vi "WaitPassTactic.vi"(6 "Tactic index in":i32, 7 "first call":bool, 8 "error in (no error)":errorcluster, 9 "Robot":refnum<class "Robot.lvclass">, 10 "Game in":refnum<class "Game.lvclass">, 11 "WaitPassTactic in":refnum<class "WaitPassTactic.lvclass">) -> (0 "error out":errorcluster, 2 "Robot out":refnum<class "Robot.lvclass">, 3 "WaitPassTactic out":refnum<class "WaitPassTactic.lvclass">)   [LabVIEW 2018, in "WaitPassTactic.lvclass"]
uses:
  WaitPassTactic.lvclass
  Robot_class/Robot.lvclass
  Game_class/Game.lvclass
  Tactic_class/Tactic.lvclass/Tactic.ctl
  Game_class/Game.lvclass/Game.ctl
  Team_class/Team.lvclass/Team.ctl
  Robot_class/Robot.lvclass/Robot.ctl
  Robot_class/tactics.ctl
  Robot_class/roles.ctl
  Skillbook_class/Skillbook.lvclass/Skillbook.ctl
  Robot_class/Read role.vi
  Skillbook_class/Read WaitBallTrajSkill.vi
  Skillbook_class/Read WaitBallKickerSkill.vi
  Skillbook_class/Read WaitBallOrientSkill.vi
  Game_class/Read OffensiveTeam.vi
  Team_class/Read OffensivePlay.vi
  Tactic_class/Read Skillbook.vi
  Robot_class/Write tactic.vi
  Ally_class/Ally.lvclass
  Skillbook_class/Skillbook.lvclass
  WaitBallTrajSkill_class/WaitBallTrajSkill.lvclass
  WaitBallKickerSkill_class/WaitBallKickerSkill.lvclass
  WaitBallOrientSkill_class/WaitBallOrientSkill.lvclass
panel:
  out "x .or. y? 2":bool
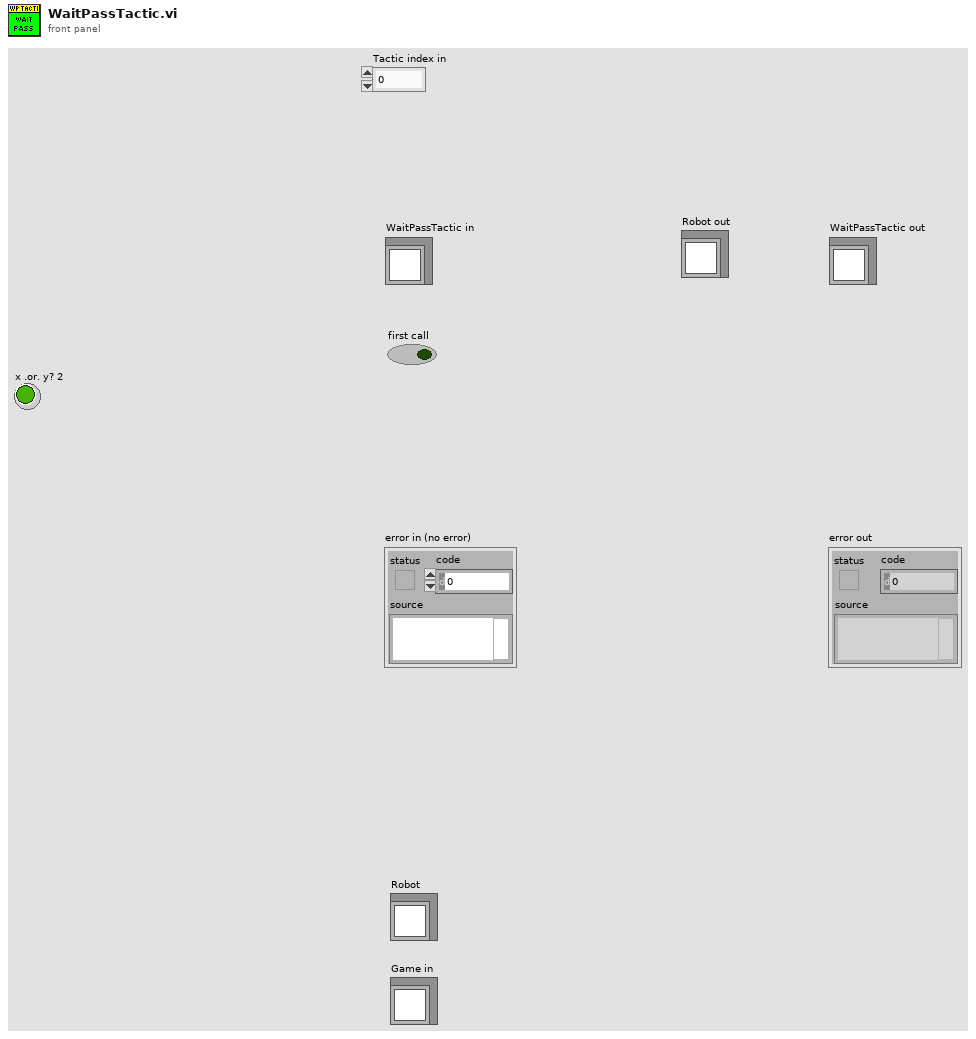
[diagram p1: front panel]
types:
  T1 = typedef "tactics.ctl" = enum16{"ReceivePassInFuturePoint", "Roller", "PrepareRollToPassRollerGoTo", "PrepareRollToPassReceiverGoTo", "WaitRoll", "PositionToRoll", "PenaltyAttacker", "PassObserver", "PenaltyDefense", "TableReceiverTactic", "Test", "DefendGoal", "Marker", "FollowAttacker", "DefendArea", "Shoot", "AttackerAimGoal", "AttackerBallOutOfField", "AttackerBlock", "AttackerStop", "Duelist", "Halt", "ZigZag", "GoTo", "Timeout", "KickToPassReceiver", "PositionToReceivePass", "WaitPass"}
  T2 = typedef "roles.ctl" = enum16{"Tabler", "TableFinalizer", "PrepareRollToPassRoller", "PrepareRollToPassReceiver", "SimplePassRoll", "SimplePassRollReceiver", "PenaltyDefense", "PreparePassReceiver 2", "PreparePassReceiver 1", "PassObserver", "Timeout", "Goto", "ZigZag", "None", "BallOutOfField", "DefenderArea", "Duelist", "AttackerStop", "FollowAttacker", "KeeperRole", "KickPenalty", "AttackerAimGoal", "AttackerBlock", "Marker", "Halt", "Shoot", "PassKicker", "PassReceiver", "TestRole", "PenaltyAttacker"}
  T3 = typedef "OffensivePlay.ctl" = enum16{"TableWithStriker", "TableWith2ndStrikerPlay", "PrepareDoublePass", "PrepareRollToPass", "SimplePass", "PreparePass", "PassToStriker", "BallOutOfField", "PassTo2ndStriker", "StopOffensive", "Prepare Penalty Enemy", "EnemyPossessionAtEnemyField", "EnemyPossesionAtOurField", "TestPlay", "PreparePenaltyAlly", "KickPenaltyAlly", "PrepareKickoffAlly", "PrepareKickoffEnemy", "IndirectEnemy", "DirectEnemy", "NormalGame", "DirectKick", "Pass", "Halt", "Timeout", "PassPlay", "PenaltyEnemy"}
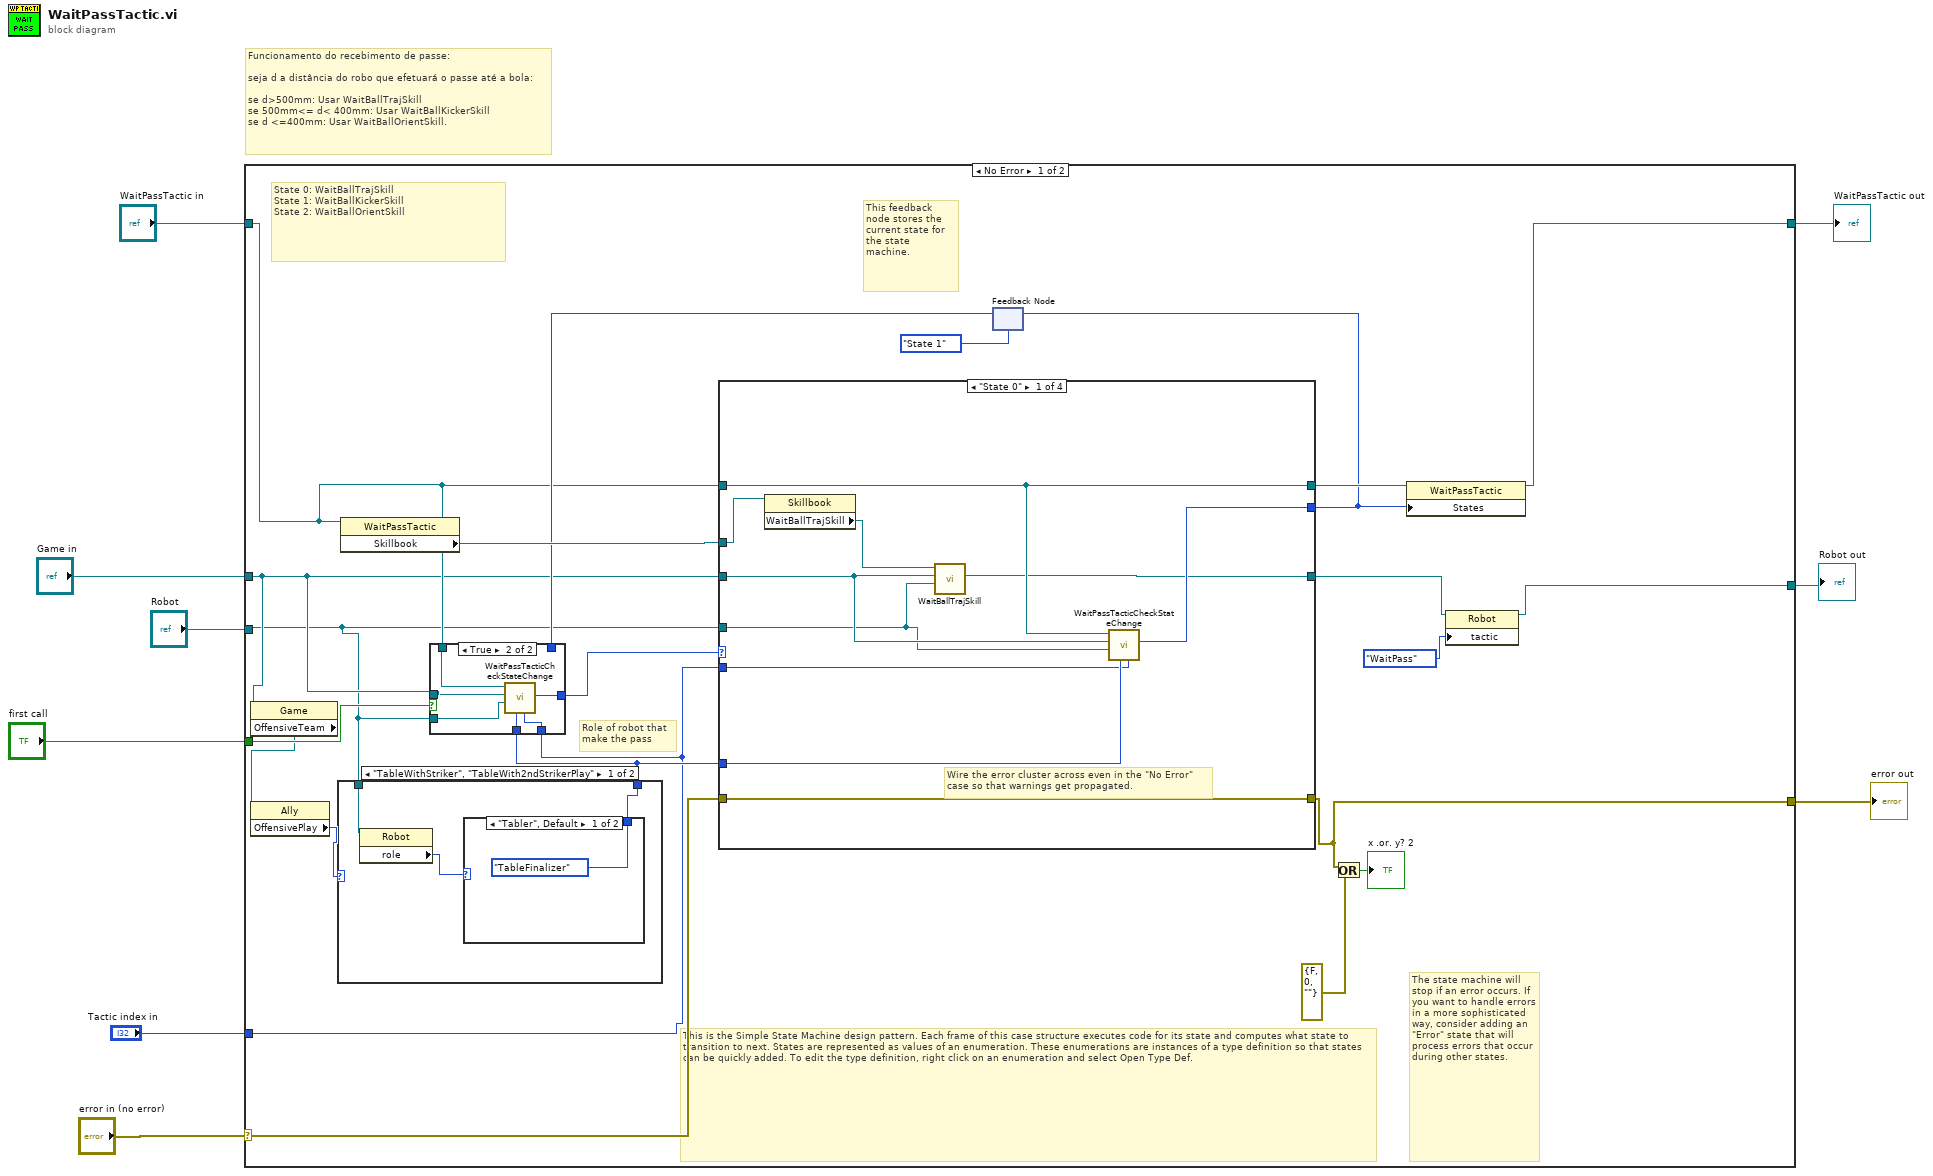
[diagram p0: block diagram]
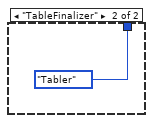
[diagram p2: hidden frame]
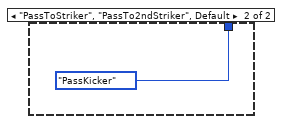
[diagram p3: hidden frame]
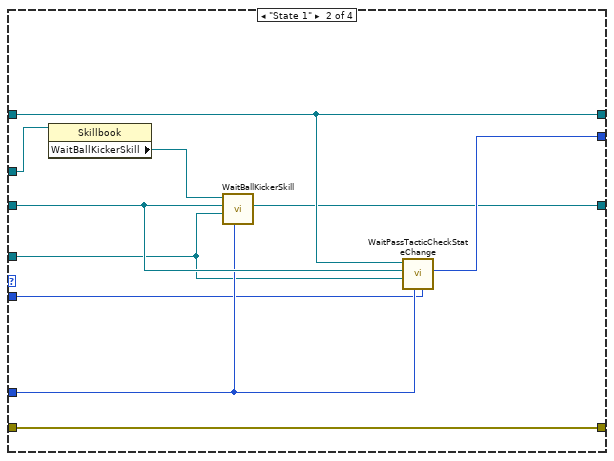
[diagram p5: hidden frame]
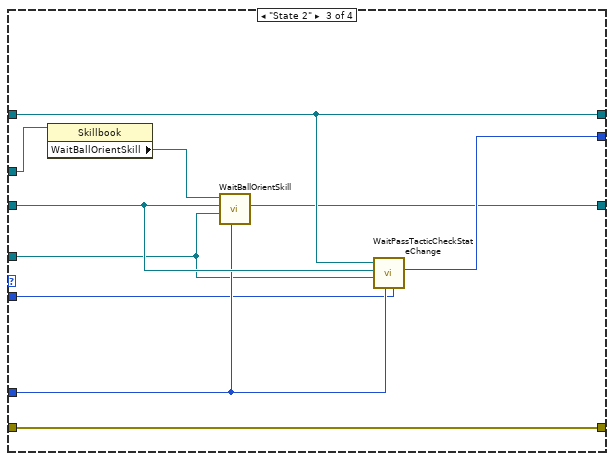
[diagram p6: hidden frame]
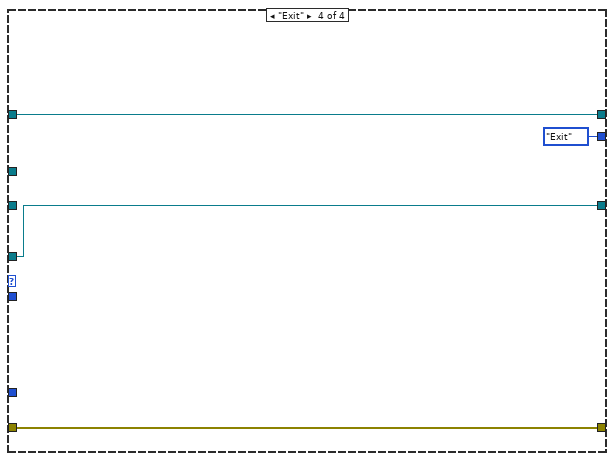
[diagram p7: hidden frame]
diagram:
  # "Funcionamento do recebimento de passe:\n\nseja d a distância do robo que efetuará o passe até a bola:\n\nse d>500mm: Usar WaitBallTrajSkill\nse 500mm<= d< 400mm: Usar WaitBallKickerSkill\nse d <=400mm: Usar WaitBallOrientSkill."
  n1 = case shown="No Error" "error in (no error)" {
    selector: "error in (no error)" -> [w20 w81]
    tunnel: [w19 w81] -> w8
    tunnel: [w17 w80] -> w6
    tunnel: "WaitPassTactic in" -> [w22 w80]
    tunnel: "Game in" -> [w15 _]
    tunnel: "Robot" -> [w12 w79]
    tunnel: [w18 w79] -> w4
    tunnel: "first call" -> [w21 _]
    tunnel: "Tactic index in" -> [w10 _]
    frame No Error {
      # "Role of robot that\nmake the pass"
      # "State 0: WaitBallTrajSkill\nState 1: WaitBallKickerSkill\nState 2: WaitBallOrientSkill"
      # "The state machine will stop if an error occurs. If you want to handle errors in a more sophisticated way, consider adding an \"Error\" state that will process errors that occur during other states."
      # "This feedback node stores the current state for the state machine."
      # "This is the Simple State Machine design pattern. Each frame of this case structure executes code for its state and computes what state to transition to next. States are represented as values of an enumeration. These enumerations are instances of a type definition so that states can be quickly added. To edit the type definition, right click on an enumeration and select Open Type Def."
      # "Wire the error cluster across even in the \"No Error\"\ncase so that warnings get propagated."
      n2 = property class="Game"(reference=w15) -> ("OffensiveTeam"=w14:refnum<class "Ally.lvclass">)  [unwired: 1 in, 2 out]
      n3 = property class="Ally"(reference=w14) -> ("OffensivePlay"=w13:T3)  [unwired: 1 in, 2 out]
      n4 = case shown="\"TableWithStriker\", \"TableWith2ndStrikerPlay\"" w13 {
        tunnel: [w32 roles."PassKicker" ("Role ofRobotThat\nmake the pass")] -> w11
        tunnel: w12 -> [w34 _]
        frame "TableWithStriker", "TableWith2ndStrikerPlay" {
          n5 = property class="Robot"(reference=w34) -> ("role"=w33:T2)  [unwired: 1 in, 2 out]
          n6 = case shown="\"Tabler\", Default" w33 {
            tunnel: [roles."TableFinalizer" ("Role ofRobotThat\nmake the pass") roles."Tabler" ("Role ofRobotThat\nmake the pass")] -> w32
            frame "Tabler", Default {
            }
            frame "TableFinalizer" {
            }
          }
        }
        frame "PassToStriker", "PassTo2ndStriker", Default {
        }
      }
      n7 = property class="WaitPassTactic"(reference=w22) -> ("Skillbook"=w30:refnum<class "Skillbook.lvclass">)  [unwired: 1 in, 2 out]
      n8 = feedback #1(enum16{"State 0", "State 1", "State 2", "Exit"}."State 1" ("States")) -> (w28:enum16{"State 0", "State 1", "State 2", "Exit"})
      n9 = case shown="True" w21 {
        tunnel: [w38 w42] -> w27
        tunnel: w28 -> [w38 _]
        tunnel: w15 -> [_ w43]
        tunnel: w22 -> [_ w44]
        tunnel: w12 -> [_ w41]
        tunnel: w11 -> [_ w40]
        tunnel: w10 -> [_ w39]
        frame False {
        }
        frame True {
          n10 = call "WaitPassTacticCheckStateChange.vi"("Tactic index in"=w39, "Role ofRobotThat\nmake the pass"=w40, "Robot in"=w41, "Game"=w43, "WaitPassTactic in"=w44) -> ("States"=w42:enum16{"State 0", "State 1", "State 2", "Exit"})  [unwired: 4 in, 2 out]
        }
      }
      n11 = case shown="\"State 0\"" w27 {
        tunnel: w20 -> [w54 w64 w74 w78]
        tunnel: [w54 w64 w74 w78] -> w19
        tunnel: w30 -> [w53 w63 w73 _]
        tunnel: w12 -> [w47 w56 w66 w75]
        tunnel: [w49 w58 w68 w75] -> w24
        tunnel: [w51 w62 w72 w77] -> w29
        tunnel: w22 -> [w51 w62 w72 w77]
        tunnel: w15 -> [w50 w59 w69 _]
        tunnel: [w52 w61 w71 enum16{"State 0", "State 1", "State 2", "Exit"}."Exit" ("States")] -> w16
        tunnel: w11 -> [w46 w57 w67 _]
        tunnel: w10 -> [w45 w55 w65 _]
        frame "State 0" {
          n12 = property class="Skillbook"(reference=w53) -> ("WaitBallTrajSkill"=w48:refnum<class "WaitBallTrajSkill.lvclass">)  [unwired: 1 in, 2 out]
          n13 = call "WaitBallTrajSkill.vi"("Robot"=w47, "Game"=w50, "WaitBallTrajSkill in"=w48) -> ("robot out"=w49:refnum<class "Robot.lvclass">)  [unwired: 6 in, 2 out]
          n14 = call "WaitPassTacticCheckStateChange.vi"("Tactic index in"=w45, "Role ofRobotThat\nmake the pass"=w46, "Robot in"=w47, "Game"=w50, "WaitPassTactic in"=w51) -> ("States"=w52:enum16{"State 0", "State 1", "State 2", "Exit"})  [unwired: 4 in, 2 out]
        }
        frame "State 1" {
          n15 = property class="Skillbook"(reference=w63) -> ("WaitBallKickerSkill"=w60:refnum<class "WaitBallKickerSkill.lvclass">)  [unwired: 1 in, 2 out]
          n16 = call "WaitBallKickerSkill.vi"("Role ofRobotThat\nmake the pass"=w57, "Robot"=w56, "Game"=w59, "WaitBallKickerSkill in"=w60) -> ("robot out"=w58:refnum<class "Robot.lvclass">)  [unwired: 5 in, 2 out]
          n17 = call "WaitPassTacticCheckStateChange.vi"("Tactic index in"=w55, "Role ofRobotThat\nmake the pass"=w57, "Robot in"=w56, "Game"=w59, "WaitPassTactic in"=w62) -> ("States"=w61:enum16{"State 0", "State 1", "State 2", "Exit"})  [unwired: 4 in, 2 out]
        }
        frame "State 2" {
          n18 = property class="Skillbook"(reference=w73) -> ("WaitBallOrientSkill"=w70:refnum<class "WaitBallOrientSkill.lvclass">)  [unwired: 1 in, 2 out]
          n19 = call "WaitBallOrientSkill.vi"("Role ofRobotThat\nmake the pass"=w67, "Robot"=w66, "Game"=w69, "WaitBallOrientSkill in"=w70) -> ("robot out"=w68:refnum<class "Robot.lvclass">)  [unwired: 5 in, 2 out]
          n20 = call "WaitPassTacticCheckStateChange.vi"("Tactic index in"=w65, "Role ofRobotThat\nmake the pass"=w67, "Robot in"=w66, "Game"=w69, "WaitPassTactic in"=w72) -> ("States"=w71:enum16{"State 0", "State 1", "State 2", "Exit"})  [unwired: 4 in, 2 out]
        }
        frame "Exit" {
        }
      }
      n21 = feedback-in #1(w16) -> ()
      n22 = Or(x=w19, y=errorcluster {"status"=FALSE, "code"=0, "source"=""}) -> (x .or. y?=→"x .or. y? 2":bool)
      n23 = property class="WaitPassTactic"(reference=w29, "States"=w16) -> (reference out=w17:refnum<class "WaitPassTactic.lvclass">)  [unwired: 1 in, 1 out]
      n24 = property class="Robot"(reference=w24, "tactic"=tactics."WaitPass") -> (reference out=w18:refnum<class "Robot.lvclass">)  [unwired: 1 in, 1 out]
    }
    frame Error {
    }
  }
  "error out" <- w8
  "WaitPassTactic out" <- w6
  "Robot out" <- w4
